vi "ANAL_DQ.vi"(8 "error in (no error)":errorcluster, 10 "State":T1=enum."ProgInit", 11 "queue In":refnum<queue>) -> (0 "error out":errorcluster, 2 "State Out":T1=enum."Idle", 4 "Exit?":bool)   [LabVIEW 2021]
uses:
  ANAL_State.ctl
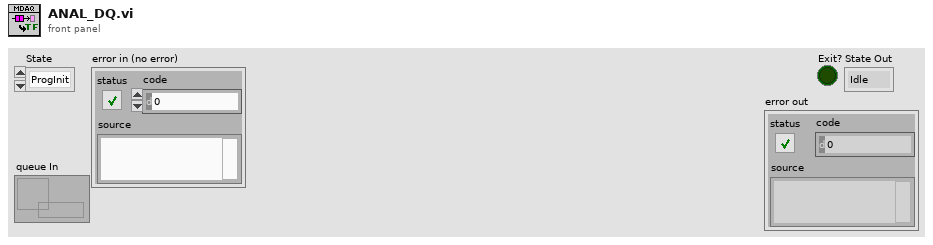
[diagram p1: front panel]
types:
  T1 = typedef "ANAL_State.ctl" = enum16{"RefreshSpectPlot", "RefreshPlotUI", "RefreshPlots", "UpdateTree", "DeriveData", "RemItem", "PrevItem", "NextItem", "Refresh", "Load File", "Idle", "ProgInit"}
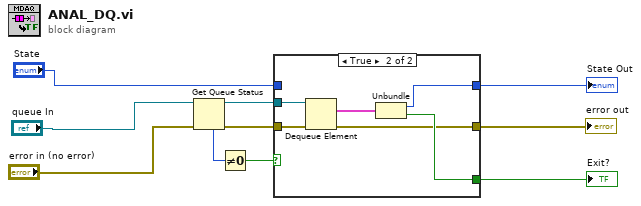
[diagram p0: block diagram]
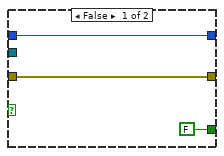
[diagram p2: hidden frame]
diagram:
  n1 = Get Queue Status(queue="queue In", error in (no error)="error in (no error)") -> (queue out=w8:refnum<queue>, error out=w6:errorcluster, # elements in queue=w9:i32)  [unwired: 1 in, 5 out]
  n2 = Not Equal To 0?(x=w9) -> (x != 0?=w10:bool)
  n3 = case shown="True" w10 {
    tunnel: w8 -> [_ w19]
    tunnel: "State" -> [w12 _]
    tunnel: [FALSE w17] -> w4
    tunnel: [w12 w16] -> w1
    tunnel: w6 -> [w11 w15]
    tunnel: [w11 w14] -> w5
    frame False {
    }
    frame True {
      n4 = Dequeue Element(queue=w19, error in (no error)=w15) -> (element=w18:cluster{"State":T1, bool}, error out=w14:errorcluster)  [unwired: 1 in, 2 out]
      n5 = Unbundle(w18) -> ("State"=w16:T1, w17:bool)
    }
  }
  "error out" <- w5
  "Exit?" <- w4
  "State Out" <- w1
